vi "Flatten.vi"(8 "error in (no error)":errorcluster, 11 "Cluster":variant) -> (0 "error out":errorcluster, 3 "String":string)   [LabVIEW 2018, in "TCPServer.lvlib"]
uses:
  TCPServer.lvlib
  <vilib>/Utility/Data Type/NI_Data Type.lvlib
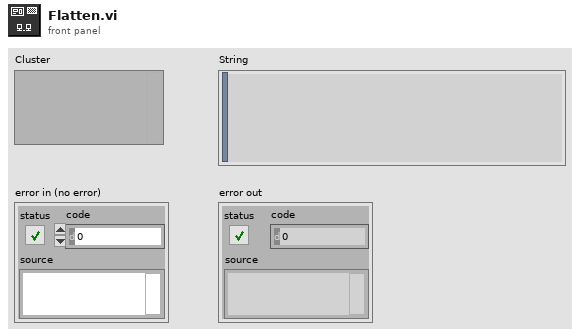
[diagram p1: front panel]
types:
  T1 = typedef "NI_Data Type.lvlib/Data Type.ctl" = enum8{"Invalid Type", "Void", "I8", "I16", "I32", "I64", "U8", "U16", "U32", "U64", "Single Float", "Double Float", "Extended Float", "Single Complex", "Double Complex", "Extended Complex", "Enum U8", "Enum U16", "Enum U32", "Enum U64", "Single Float With Unit", "Double Float With Unit", "Extended Float With Unit", "Single Complex with Unit", "Double Complex with Unit", "Extended Complex with Unit", "Boolean", "String", "Path", "Picture", "Tag", "Array", "Cluster", "Variant", "LV Variant", "Waveform", "Timestamp", "Digital Waveform", "Digital Data", "ExpressData", "Refnum", "External Data", "VI", "Poly VI", "LabVIEW Class Instance", "Fixed Point", "Set Collection", "Map Collection"}
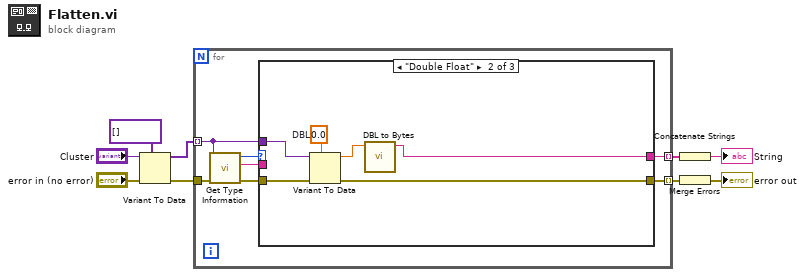
[diagram p0: block diagram]
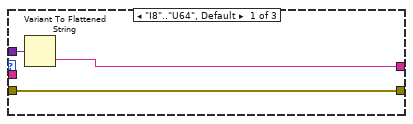
[diagram p2: hidden frame]
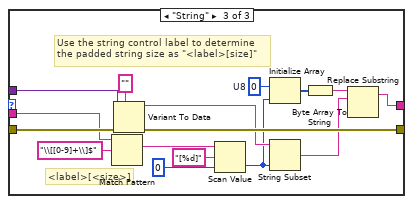
[diagram p3: hidden frame]
diagram:
  n1 = Variant To Data(error in="error in (no error)", type=variant[] [], Variant="Cluster") -> (data=w7:variant[], error out=w6:errorcluster)
  n2 = for {
    tunnel: w7 -> [w13] mode=indexing
    tunnel: w6 -> [w16]
    tunnel: [w14] -> w4 mode=indexing
    tunnel: [w11] -> w2 mode=indexing
    n3 = call <vilib>:"Get Type Information.vi"("error in (no error)"=w16, "variant"=w13) -> ("error out"=w15:errorcluster, "name"=w10:string, "type"=w12:T1)  [unwired: 5 in, 2 out]
    n4 = case shown="\"Double Float\"" w12 {
      tunnel: w15 -> [w19 w25 w41]
      tunnel: [w19 w24 w40] -> w14
      tunnel: w13 -> [w18 w23 w39]
      tunnel: [w17 w20 w30] -> w11
      tunnel: w10 -> [_ _ w37]
      frame "I8".."U64", Default {
        n5 = Variant To Flattened String(Variant=w18) -> (data string=w17:string)  [unwired: 1 out]
      }
      frame "Double Float" {
        w22 = 0.0  # DBL
        n6 = Variant To Data(error in=w25, type=w22, Variant=w23) -> (data=w21:dbl, error out=w24:errorcluster)
        n7 = call "DBL to Bytes.vi"("Numeric"=w21) -> ("ASIST DBL"=w20:string)  [unwired: 10 in]
      }
      frame "String" {
        w35 = u8 0  # U8
        # "Use the string control label to determine\nthe padded string size as \"<label>[size]\""
        # "<label>[<size>]"
        n8 = Match Pattern(string=w37, regular expression="\\[[0-9]+\\]$") -> (match substring=w29:string)  [unwired: 1 in, 3 out]
        n9 = Variant To Data(error in=w41, type="", Variant=w39) -> (data=w31:string, error out=w40:errorcluster)
        n10 = Scan Value(string=w29, format string="[%d]", default (0 dbl)=0 ("default value 1")) -> (value=w27:i32)  [unwired: 1 out]
        n11 = Initialize Array(w35, w27) -> (w34:u8[])
        n12 = String Subset(string=w31, length (rest)=w27) -> (substring=w32:string)  [unwired: 1 in]
        n13 = Byte Array To String(unsigned byte array=w34) -> (string=w33:string)
        n14 = Replace Substring(4:w32, 5:w33) -> (1:w30:string)  [unwired: 2 in, 1 out]
      }
    }
  }
  n15 = Concatenate Strings(w2) -> (→"String":string)
  n16 = Merge Errors(w4) -> (→"error out":errorcluster)
